vi "16CH Relay Array.vi"(11 "Relays In":bool[](array[boolean])) -> (1 "Relays9-16":bool[](array[boolean]), 2 "Relays1-8":bool[](array[boolean]), 3 "Relays1-16":bool[](array[boolean]))   [LabVIEW 2020]
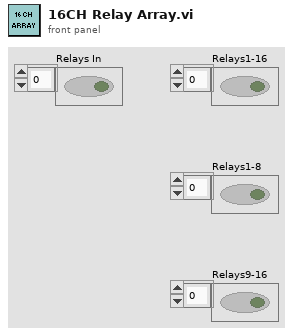
[diagram p1: front panel]
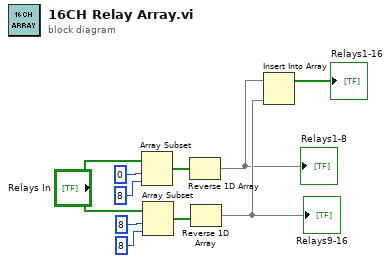
[diagram p0: block diagram]
diagram:
  n1 = Array Subset(array="Relays In", index=0, length=8) -> (w6:bool[])
  n2 = Array Subset(array="Relays In", index=8, length=8) -> (w7:bool[])
  n3 = Reverse 1D Array(array=w6) -> (reversed array=w8:bool[])
  "Relays1-8" <- w8
  n4 = Reverse 1D Array(array=w7) -> (reversed array=w9:bool[])
  "Relays9-16" <- w9
  n5 = Insert Into Array(array=w8, new element=w9) -> (→"Relays1-16":bool[])  [unwired: 1 in]
